vi "Untitled 2.vi"(6 "Axis":enum16{"X", "Y", "X+Y"}(ring), 7 "error IN":errorcluster, 10 "Data IN":T1={"App State"="", "Connect "=FALSE, "phandle out"=0, "Axis"=[], "S ramp"=30.0, "Acceleration"=100000.0, "Initial Speed"=10.0, "Normal Open / Close"=enum."Close", "Deceleration"=100000.0, "Creep"=30.0, "Speed"=1000.0, "X Axis"={"Operating State"="", "Current Position"=0.0, "Current Speed"=0.0, "Axis State"=0, "Angle"=0.0}, "Y Axis"={"Operating State"="", "Current Position"=0.0, "Current Speed"=0.0, "Axis State"=0, "Angle"=0.0}, "Distance"=0.0, "Direct of movement"=enum."Forward", "Move Method"=enum."Continue", "Move Mode"=enum."Relative", "Angle"=enum."0", "Times"=0, "Start Time"=0.0, "Step Flag"=FALSE, "x  dist"=[], "y dist"=[], "x angle array"=[], "y angle array"=[], "index"=0.0, "big motion angle"=0.0, "big angle"=[]}) -> (0 "error out":errorcluster, 3 "Data OUT":T1={"App State"="", "Connect "=FALSE, "phandle out"=0, "Axis"=[], "S ramp"=30.0, "Acceleration"=100000.0, "Initial Speed"=10.0, "Normal Open / Close"=enum."Close", "Deceleration"=100000.0, "Creep"=30.0, "Speed"=1000.0, "X Axis"={"Operating State"="", "Current Position"=0.0, "Current Speed"=0.0, "Axis State"=0, "Angle"=0.0}, "Y Axis"={"Operating State"="", "Current Position"=0.0, "Current Speed"=0.0, "Axis State"=0, "Angle"=0.0}, "Distance"=0.0, "Direct of movement"=enum."Forward", "Move Method"=enum."Continue", "Move Mode"=enum."Relative", "Angle"=enum."0", "Times"=0, "Start Time"=0.0, "Step Flag"=FALSE, "x  dist"=[], "y dist"=[], "x angle array"=[], "y angle array"=[], "index"=0.0, "big motion angle"=0.0, "big angle"=[]})   [LabVIEW 2015]
uses:
  Typedef/Data2.ctl
  zauxdll-2014/zauxdll.lvlib
panel:
  out "y angle array":i32[][](array[numeric])
  out "x angle array":i32[][](array[numeric])
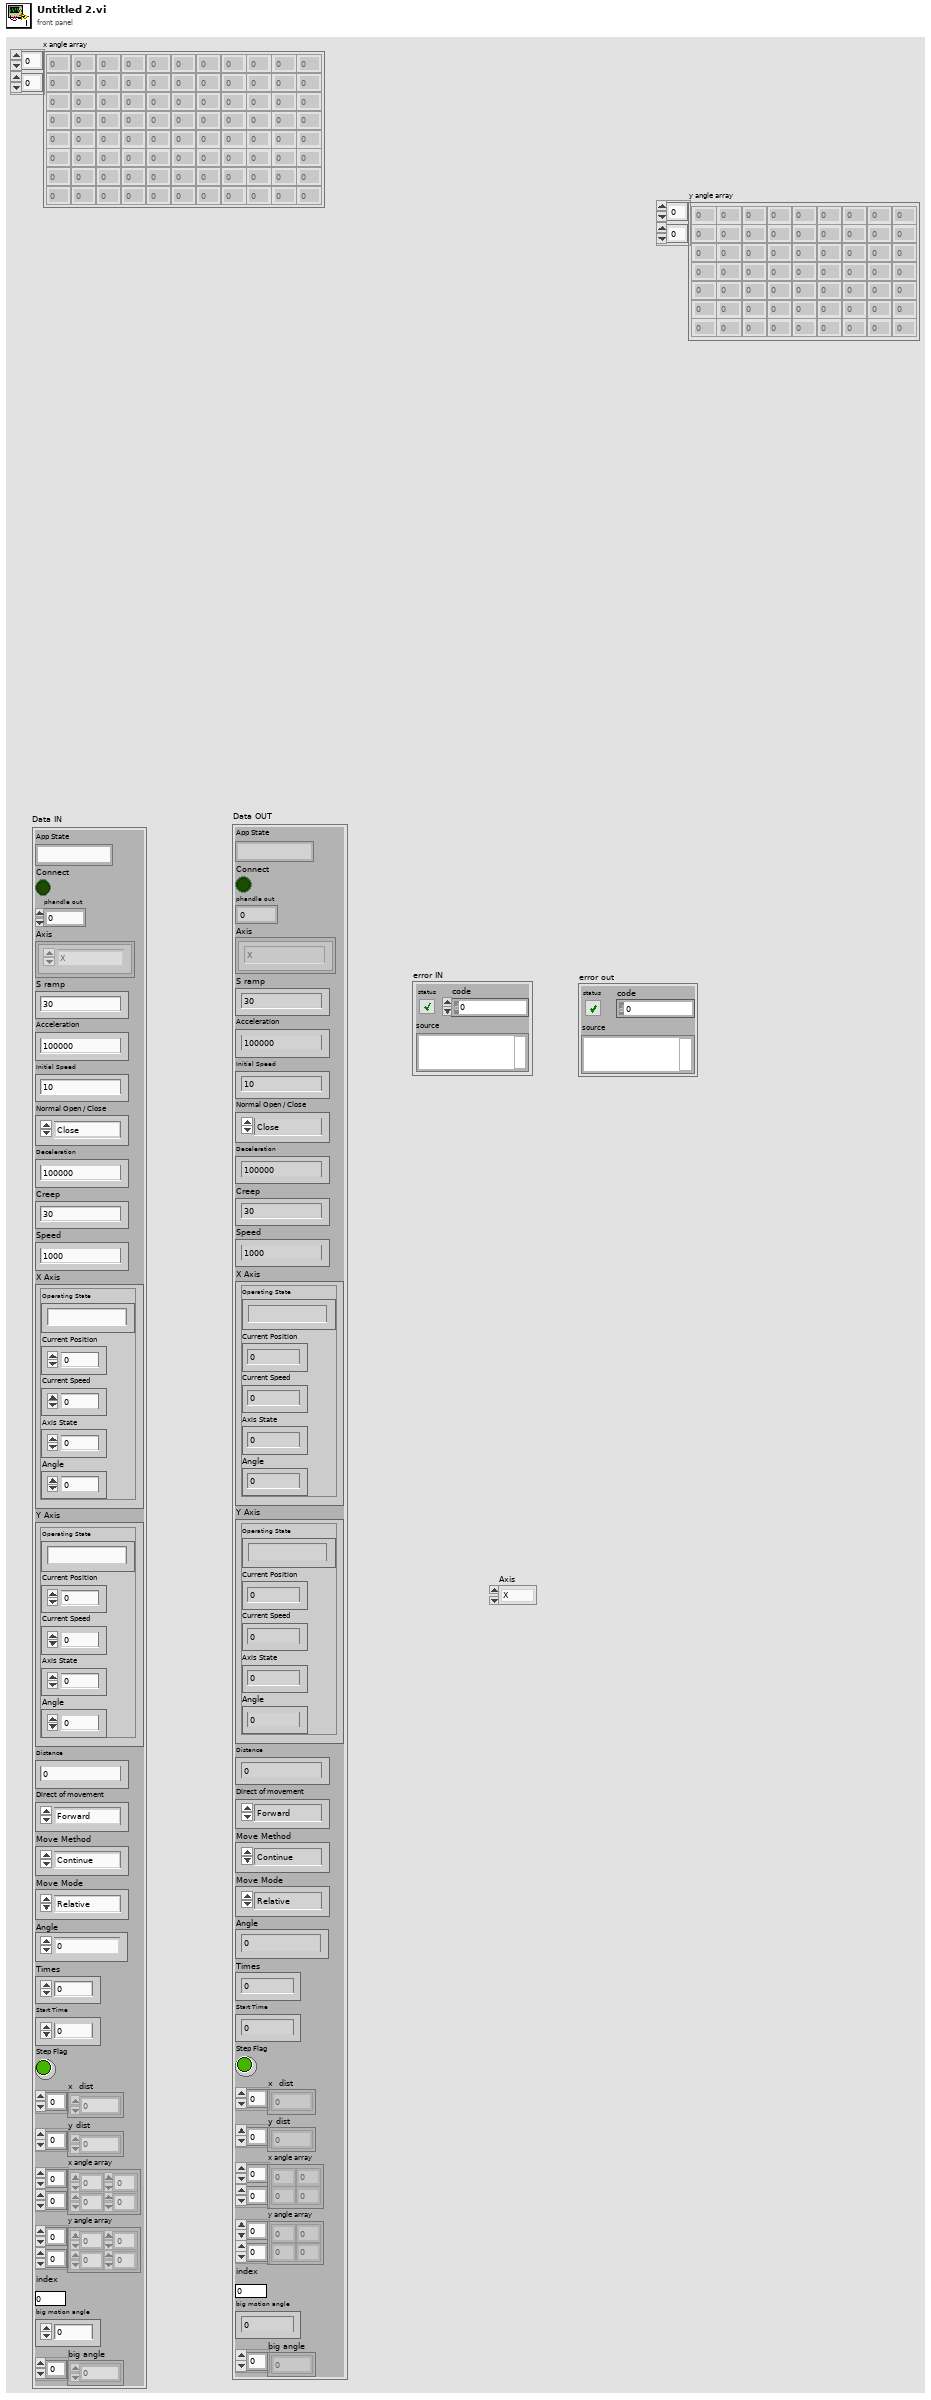
[diagram p1: front panel]
types:
  T1 = typedef "Data2.ctl" = cluster{"App State":string, "Connect ":bool, "phandle out":u32, "Axis":enum16{"X", "Y", "X+Y"}[], "S ramp":dbl, "Acceleration":dbl, "Initial Speed":dbl, "Normal Open / Close":enum16{"Open", "Close"}, "Deceleration":dbl, "Creep":dbl, "Speed":dbl, "X Axis":cluster{"Operating State":string, "Current Position":dbl, "Current Speed":dbl, "Axis State":i32, "Angle":dbl}, "Y Axis":cluster{"Operating State":string, "Current Position":dbl, "Current Speed":dbl, "Axis State":i32, "Angle":dbl}, "Distance":dbl, "Direct of movement":enum16{"Forward", "Backward"}, "Move Method":enum16{"Continue", "Inching"}, "Move Mode":enum16{"Relative", "Absolute"}, "Angle":enum32{"0", "1", "10", "30", "34", "60", "90", "180", "-1", "-10"}, "Times":i32, "Start Time":dbl, "Step Flag":bool, "x  dist":dbl[], "y dist":dbl[], "x angle array":i32[][], "y angle array":i32[][], "index":dbl, "big motion angle":dbl, "big angle":dbl[]}
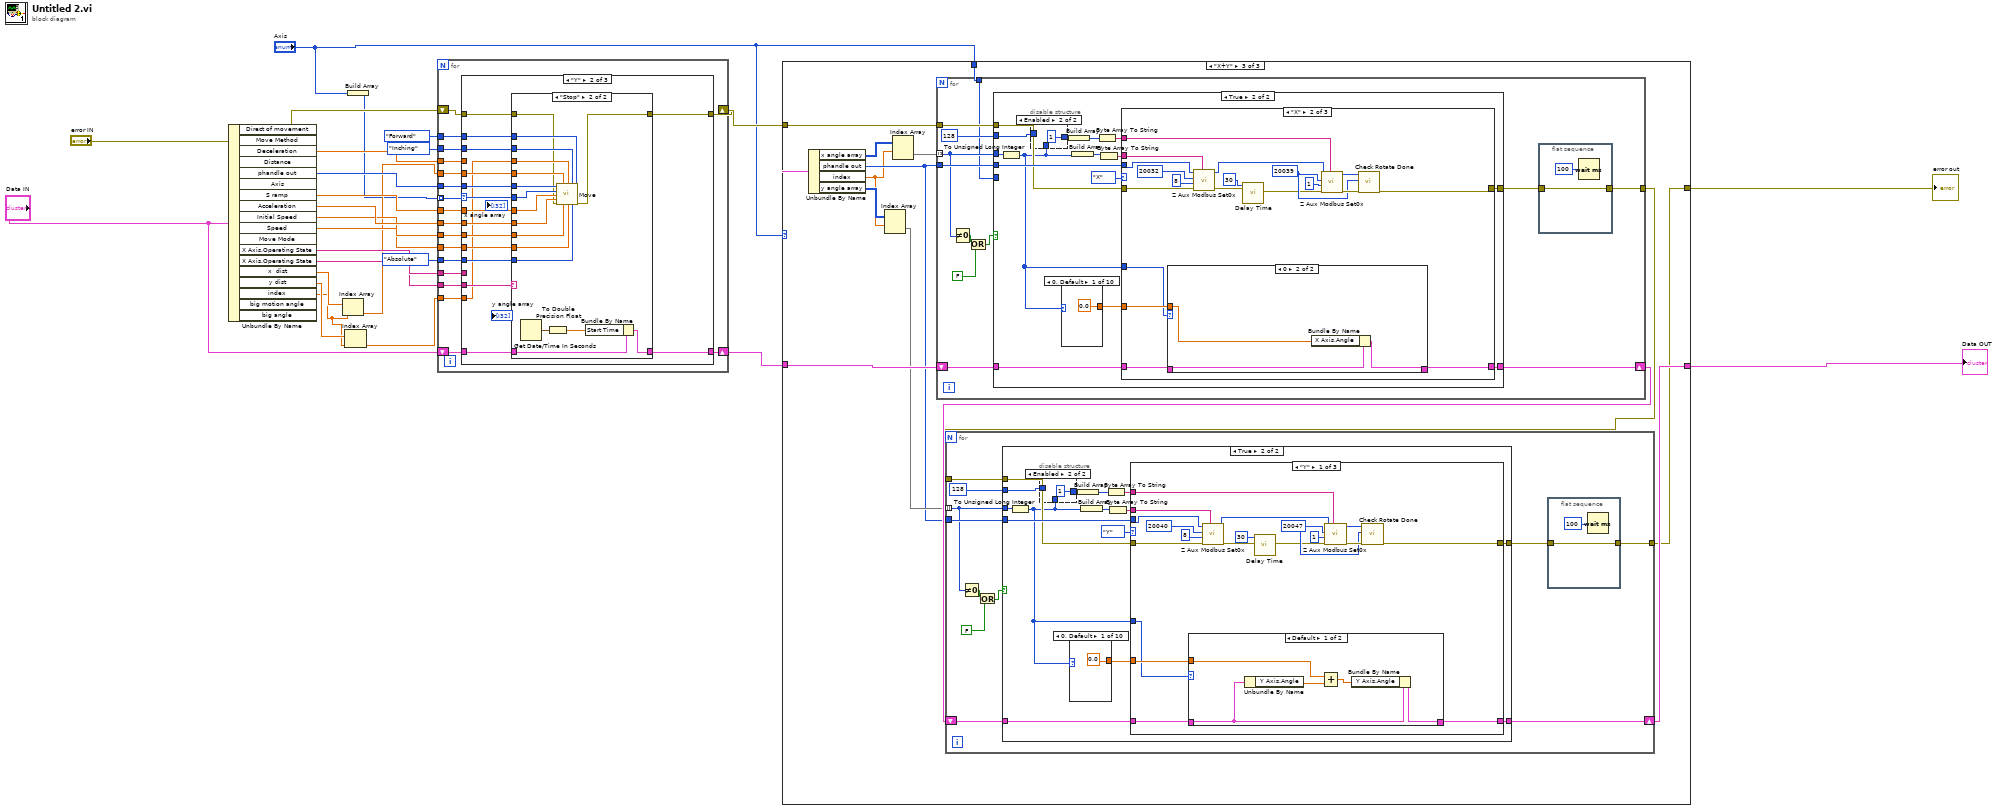
[diagram p0: block diagram]
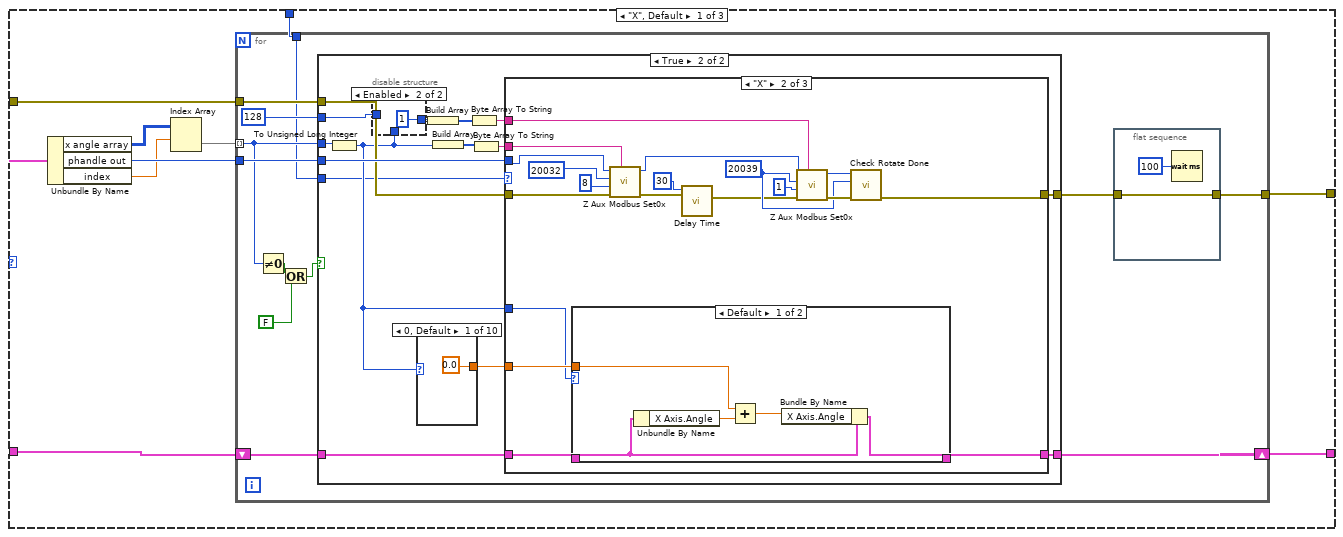
[diagram p2: hidden frame]
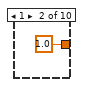
[diagram p4: hidden frame]
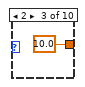
[diagram p5: hidden frame]
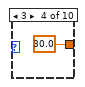
[diagram p6: hidden frame]
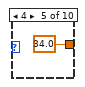
[diagram p7: hidden frame]
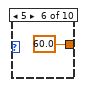
[diagram p8: hidden frame]
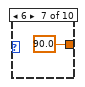
[diagram p9: hidden frame]
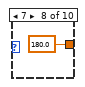
[diagram p10: hidden frame]
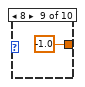
[diagram p11: hidden frame]
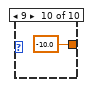
[diagram p12: hidden frame]
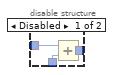
[diagram p13: hidden frame]
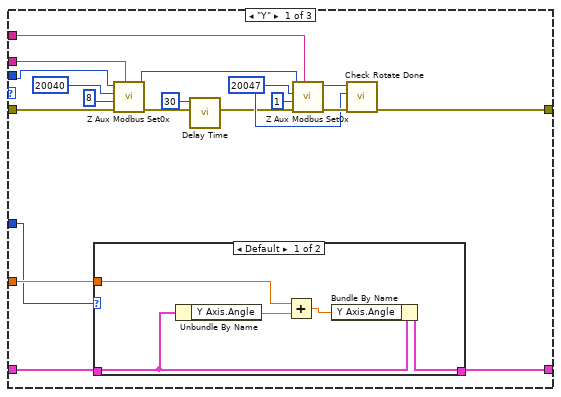
[diagram p14: hidden frame]
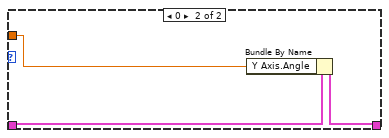
[diagram p15: hidden frame]
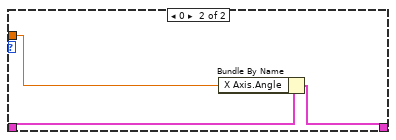
[diagram p16: hidden frame]
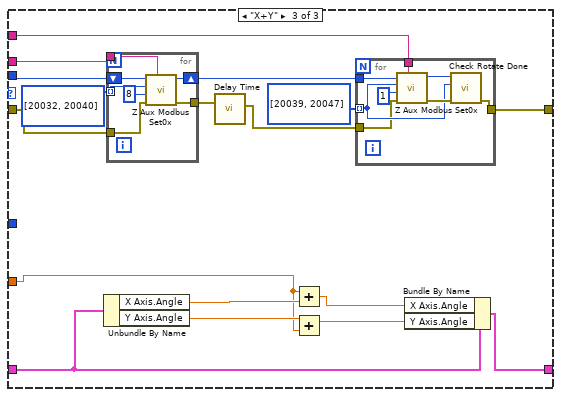
[diagram p17: hidden frame]
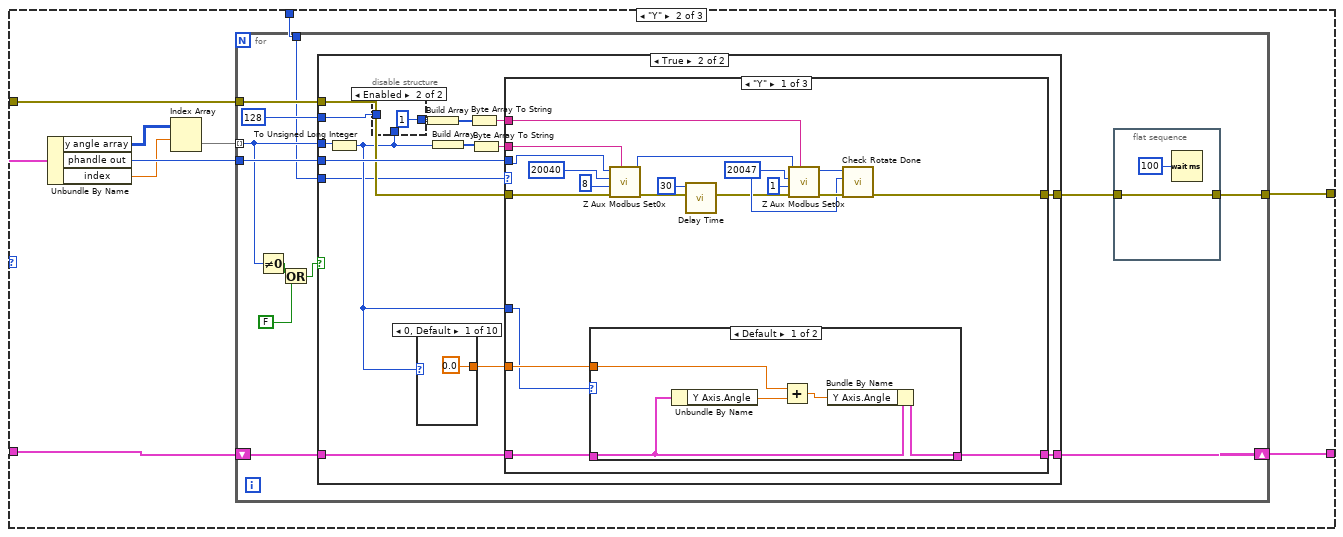
[diagram p18: hidden frame]
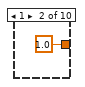
[diagram p20: hidden frame]
diagram:
  n1 = Unbundle By Name("Data IN") -> ("Deceleration"=w19:dbl, "phandle out"=w24:u32, "S ramp"=w23:dbl, "Acceleration"=w22:dbl, "Initial Speed"=w21:dbl, "Speed"=w20:dbl, "X Axis.Operating State"=w18:string, "X Axis.Operating State"=w17:string, "x  dist"=w10:dbl[], "y dist"=w3:dbl[], "index"=w2:dbl)  [unwired: 7 out]
  n2 = Index Array(array=w10, index=w2) -> (element=w6:dbl)
  n3 = Index Array(array=w3, index=w2) -> (element=w1:dbl)
  n4 = Build Array("Axis") -> (w5:enum16{"X", "Y", "X+Y"}[])
  n5 = for {
    tunnel: w24 -> [w42]
    tunnel: w23 -> [w41]
    tunnel: w22 -> [w40]
    tunnel: w21 -> [w39]
    tunnel: w20 -> [w38]
    tunnel: enum16{"Continue", "Inching"}."Inching" ("Move Method") -> [w37]
    tunnel: w19 -> [w36]
    tunnel: w5 -> [w35] mode=indexing
    tunnel: w6 -> [w34]
    tunnel: enum16{"Forward", "Backward"}."Forward" ("Direct of movement") -> [w33]
    tunnel: enum16{"Relative", "Absolute"}."Absolute" ("Move Mode") -> [w32]
    tunnel: w18 -> [w31]
    tunnel: w17 -> [w30]
    shift-right: [w28] -> w14
    shift-left: "Data IN" -> [w29]
    shift-right: [w26] -> w13
    shift-left: "error IN" -> [w27]
    tunnel: w1 -> [w25]
    n6 = case shown="\"Y\"" w35 {
      selector: w35 -> [w51 w87 _]
      tunnel: w42 -> [w58 w93 w134]
      tunnel: w41 -> [w57 w92 w133]
      tunnel: w40 -> [w56 w91 w132]
      tunnel: w39 -> [w55 w90 w131]
      tunnel: w38 -> [w54 w89 w130]
      tunnel: w37 -> [w53 w88 w129]
      tunnel: w36 -> [w52 _ w128]
      tunnel: w34 -> [w49 w85 w115]
      tunnel: w33 -> [w50 w86 w127]
      tunnel: w32 -> [w48 w84 w126]
      tunnel: w31 -> [w47 _ w125]
      tunnel: w30 -> [_ w83 w123]
      tunnel: w29 -> [w46 w82 w119]
      tunnel: [w45 w81 w118] -> w28
      tunnel: w27 -> [w44 w80 w117]
      tunnel: [w43 w79 w116] -> w26
      tunnel: w25 -> [_ w78 w114]
      frame "X", Default {
        n7 = case shown="\"Stop\"" w47 {
          tunnel: w58 -> [_ w77]
          tunnel: w57 -> [_ w76]
          tunnel: w56 -> [_ w75]
          tunnel: w55 -> [_ w74]
          tunnel: w54 -> [_ w73]
          tunnel: w53 -> [_ w72]
          tunnel: w52 -> [_ w71]
          tunnel: w51 -> [_ w70]
          tunnel: w50 -> [_ w69]
          tunnel: w49 -> [_ w68]
          tunnel: w48 -> [_ w67]
          tunnel: w46 -> [w60 w66]
          tunnel: [w60 w65] -> w45
          tunnel: w44 -> [w59 w62]
          tunnel: [w59 w61] -> w43
          frame "False", Default {
          }
          frame "Stop" {
            n8 = Get Date/Time In Seconds() -> (seconds since 1Jan1904=w64:timestamp)
            n9 = call "Move.vi"("handle"=w77, "Distance"=w68, "Decel"=w71, "Move Method"=w72, "Direct of movement"=w69, "Axis"=w70, "Sramp"=w76, "Accel"=w75, "error in (no error)"=w62, "Lspeed"=w74, "Speed"=w73, "Move Mode"=w67) -> ("error out"=w61:errorcluster)  [unwired: 3 in]
            n10 = To Double Precision Float(number=w64) -> (double precision float=w63:dbl)
            n11 = Bundle By Name(cluster=w66, "Start Time"=w63) -> (w65:T1)
          }
        }
      }
      frame "Y" {
        n12 = case shown="\"Stop\"" w83 {
          tunnel: w93 -> [_ w112]
          tunnel: w92 -> [_ w111]
          tunnel: w91 -> [_ w110]
          tunnel: w90 -> [_ w109]
          tunnel: w89 -> [_ w108]
          tunnel: w88 -> [_ w107]
          tunnel: w78 -> [_ w106]
          tunnel: w87 -> [_ w105]
          tunnel: w86 -> [_ w104]
          tunnel: w85 -> [_ w103]
          tunnel: w84 -> [_ w102]
          tunnel: w82 -> [w95 w99]
          tunnel: [w95 w98] -> w81
          tunnel: w80 -> [w94 w97]
          tunnel: [w94 w96] -> w79
          frame "False", Default {
          }
          frame "Stop" {
            n13 = Get Date/Time In Seconds() -> (seconds since 1Jan1904=w101:timestamp)
            n14 = To Double Precision Float(number=w101) -> (double precision float=w100:dbl)
            n15 = call "Move.vi"("handle"=w112, "Distance"=w103, "Decel"=w106, "Move Method"=w107, "Direct of movement"=w104, "Axis"=w105, "Sramp"=w111, "Accel"=w110, "error in (no error)"=w97, "Lspeed"=w109, "Speed"=w108, "Move Mode"=w102) -> ("error out"=w96:errorcluster)  [unwired: 3 in]
            n16 = Bundle By Name(cluster=w99, "Start Time"=w100) -> (w98:T1)
          }
        }
      }
      frame "X+Y" {
        w124 = "Stop" ("y")
        n17 = Build Array(w115, w114) -> (w113:dbl[])
        n18 = Equal?(x=w125, y=w124) -> (x = y?=w122:bool)
        n19 = Equal?(x=w124, y=w123) -> (x = y?=w120:bool)
        n20 = And(x=w122, y=w120) -> (x .and. y?=w121:bool)
        n21 = case shown="True" w121 {
          tunnel: w134 -> [_ w153]
          tunnel: w133 -> [_ w152]
          tunnel: w132 -> [_ w151]
          tunnel: w131 -> [_ w150]
          tunnel: w130 -> [_ w149]
          tunnel: w129 -> [_ w148]
          tunnel: w128 -> [_ w147]
          tunnel: w113 -> [_ w145]
          tunnel: w127 -> [_ w144]
          tunnel: w126 -> [_ w143]
          tunnel: w119 -> [w136 w142]
          tunnel: [w136 w141] -> w118
          tunnel: w117 -> [w135 w138]
          tunnel: [w135 w137] -> w116
          frame False {
          }
          frame True {
            n22 = Get Date/Time In Seconds() -> (seconds since 1Jan1904=w140:timestamp)
            n23 = To Double Precision Float(number=w140) -> (double precision float=w139:dbl)
            n24 = for {
              tunnel: w153 -> [w166]
              tunnel: w152 -> [w165]
              tunnel: w151 -> [w164]
              tunnel: w150 -> [w163]
              tunnel: w149 -> [w162]
              tunnel: w148 -> [w161]
              tunnel: w147 -> [w160]
              tunnel: i32[] [0, 1] -> [w159] mode=indexing
              tunnel: w145 -> [w158] mode=indexing
              tunnel: w144 -> [w157]
              tunnel: w143 -> [w156]
              tunnel: w138 -> [w155]
              tunnel: [w154] -> w137
              n25 = call "Move.vi"("handle"=w166, "Distance"=w158, "Decel"=w160, "Move Method"=w161, "Direct of movement"=w157, "Axis"=w159, "Sramp"=w165, "Accel"=w164, "error in (no error)"=w155, "Lspeed"=w163, "Speed"=w162, "Move Mode"=w156) -> ("error out"=w154:errorcluster)  [unwired: 3 in]
            }
            n26 = Bundle By Name(cluster=w142, "Start Time"=w139) -> (w141:T1)
          }
        }
      }
    }
  }
  n27 = case shown="\"X+Y\"" "Axis" {
    tunnel: w14 -> [w173 w313 w454]
    tunnel: w13 -> [w172 w312 w458]
    tunnel: [w171 w311 w450] -> w12
    tunnel: [w170 w310 w452] -> w11
    tunnel: "Axis" -> [w169 w309 w457]
    frame "X", Default {
      n28 = Unbundle By Name(w173) -> ("x angle array"=w168:i32[][], "phandle out"=w175:u32, "index"=w167:dbl)
      n29 = Index Array(array=w168, index (row)=w167) -> (element=w174:i32[])  [unwired: 1 in]
      n30 = for {
        tunnel: w175 -> [w183]
        tunnel: w172 -> [w187]
        tunnel: w174 -> [w182] mode=indexing
        shift-right: [w184] -> w170
        shift-left: w173 -> [w185]
        tunnel: [w178] -> w171
        tunnel: w169 -> [w176]
        n31 = Not Equal To 0?(x=w182) -> (x != 0?=w180:bool)
        n32 = Or(x=w180, y=FALSE) -> (x .or. y?=w181:bool)
        n33 = case shown="True" w181 {
          tunnel: w183 -> [_ w206]
          tunnel: w187 -> [w191 w205]
          tunnel: u32 128 -> [_ w204]
          tunnel: w185 -> [w190 w198]
          tunnel: w182 -> [_ w197]
          tunnel: [w190 w196] -> w184
          tunnel: [w191 w195] -> w179
          tunnel: w176 -> [_ w192]
          frame False {
          }
          frame True {
            n34 = To Unsigned Long Integer(number=w197) -> (unsigned 32bit integer=w193:u32)
            n35 = disable-structure shown="Enabled" {
              disable-tunnel: w204 -> [w219 _]
              disable-tunnel: [w218 u32 1] -> w203
              disable-tunnel: w193 -> [w217 _]
              frame Disabled {
                n36 = Add(x=w219, y=w217) -> (x+y=w218:u32)
              }
              frame Enabled {
              }
            }
            n37 = case shown="0, Default" w193 {
              tunnel: [0.0 1.0 10.0 30.0 34.0 60.0 90.0 180.0 -1.0 -10.0] -> w199
              frame 0, Default {
              }
              frame 1 {
              }
              frame 2 {
              }
              frame 3 {
              }
              frame 4 {
              }
              frame 5 {
              }
              frame 6 {
              }
              frame 7 {
              }
              frame 8 {
              }
              frame 9 {
              }
            }
            n38 = Build Array(w203) -> (w202:u32[])
            n39 = Build Array(w193) -> (w194:u32[])
            n40 = Byte Array To String(unsigned byte array=w202) -> (string=w201:string)
            n41 = Byte Array To String(unsigned byte array=w194) -> (string=w200:string)
            n42 = case shown="\"X\"" w192 {
              tunnel: w206 -> [w236 w263 w290]
              tunnel: w201 -> [w237 w264 w291]
              tunnel: w200 -> [w235 w262 w289]
              tunnel: w205 -> [w230 w257 w286]
              tunnel: [w225 w252 w282] -> w195
              tunnel: w198 -> [w224 w251 w279]
              tunnel: [w223 w250 w278] -> w196
              tunnel: w199 -> [w222 w249 w275]
              tunnel: w193 -> [w221 w248 _]
              frame "Y" {
                w231 = u16 20047 ("start")
                n43 = case shown="Default" w221 {
                  tunnel: w224 -> [w244 w247]
                  tunnel: [w243 w246] -> w223
                  tunnel: w222 -> [w240 w245]
                  frame Default {
                    n44 = Unbundle By Name(w244) -> ("Y Axis.Angle"=w241:dbl)
                    n45 = Add(x=w240, y=w241) -> (x+y=w242:dbl)
                    n46 = Bundle By Name(cluster=w244, "Y Axis.Angle"=w242) -> (w243:T1)
                  }
                  frame 0 {
                    n47 = Bundle By Name(cluster=w247, "Y Axis.Angle"=w245) -> (w246:T1)
                  }
                }
                n48 = call "Z Aux Modbus Set0x.vi"("pdata"=w235, "error in (no error)"=w230, "inum"=u16 8, "start"=u16 20040, "handle"=w236) -> ("error out"=w228:errorcluster, "handle out"=w229:u32)  [unwired: 3 in, 2 out]
                n49 = call "Delay Time.vi"("error in (no error)"=w228, "Delay(ms)"=u32 30) -> ("error out"=w226:errorcluster)  [unwired: 9 in]
                n50 = call "Z Aux Modbus Set0x.vi"("pdata"=w237, "error in (no error)"=w226, "inum"=u16 1, "start"=w231, "handle"=w229) -> ("error out"=w239:errorcluster, "handle out"=w238:u32)  [unwired: 3 in, 2 out]
                n51 = call "Check Rotate Done.vi"("error in (no error)"=w239, "start"=w231, "phandle in"=w238) -> ("error out"=w225:errorcluster)  [unwired: 8 in]
              }
              frame "X" {
                w258 = u16 20039 ("start")
                n52 = case shown="Default" w248 {
                  tunnel: w251 -> [w271 w274]
                  tunnel: [w270 w273] -> w250
                  tunnel: w249 -> [w267 w272]
                  frame Default {
                    n53 = Unbundle By Name(w271) -> ("X Axis.Angle"=w269:dbl)
                    n54 = Add(x=w267, y=w269) -> (x+y=w268:dbl)
                    n55 = Bundle By Name(cluster=w271, "X Axis.Angle"=w268) -> (w270:T1)
                  }
                  frame 0 {
                    n56 = Bundle By Name(cluster=w274, "X Axis.Angle"=w272) -> (w273:T1)
                  }
                }
                n57 = call "Z Aux Modbus Set0x.vi"("pdata"=w262, "error in (no error)"=w257, "inum"=u16 8, "start"=u16 20032, "handle"=w263) -> ("error out"=w255:errorcluster, "handle out"=w256:u32)  [unwired: 3 in, 2 out]
                n58 = call "Delay Time.vi"("error in (no error)"=w255, "Delay(ms)"=u32 30) -> ("error out"=w253:errorcluster)  [unwired: 9 in]
                n59 = call "Z Aux Modbus Set0x.vi"("pdata"=w264, "error in (no error)"=w253, "inum"=u16 1, "start"=w258, "handle"=w256) -> ("error out"=w266:errorcluster, "handle out"=w265:u32)  [unwired: 3 in, 2 out]
                n60 = call "Check Rotate Done.vi"("error in (no error)"=w266, "start"=w258, "phandle in"=w265) -> ("error out"=w252:errorcluster)  [unwired: 8 in]
              }
              frame "X+Y" {
                n61 = Unbundle By Name(w279) -> ("X Axis.Angle"=w281:dbl, "Y Axis.Angle"=w280:dbl)
                n62 = for {
                  tunnel: w289 -> [w305]
                  shift-right: [w304] -> w284
                  shift-left: w290 -> [w306]
                  tunnel: i32[] [20032, 20040] -> [w302] mode=indexing
                  tunnel: w286 -> [w301]
                  tunnel: [w300] -> w285
                  n63 = call "Z Aux Modbus Set0x.vi"("pdata"=w305, "error in (no error)"=w301, "inum"=u16 8, "start"=w302, "handle"=w306) -> ("error out"=w300:errorcluster, "handle out"=w304:u32)  [unwired: 3 in, 2 out]
                }
                n64 = call "Delay Time.vi"("error in (no error)"=w285) -> ("error out"=w283:errorcluster)  [unwired: 10 in]
                n65 = Add(x=w275, y=w281) -> (x+y=w277:dbl)
                n66 = Add(x=w280, y=w275) -> (x+y=w276:dbl)
                n67 = for {
                  tunnel: w291 -> [w297]
                  tunnel: w284 -> [w296]
                  tunnel: i32[] [20039, 20047] -> [w294] mode=indexing
                  tunnel: w283 -> [w293]
                  tunnel: [w292] -> w282
                  n68 = call "Z Aux Modbus Set0x.vi"("pdata"=w297, "error in (no error)"=w293, "inum"=u16 1, "start"=w294, "handle"=w296) -> ("error out"=w299:errorcluster, "handle out"=w298:u32)  [unwired: 3 in, 2 out]
                  n69 = call "Check Rotate Done.vi"("error in (no error)"=w299, "start"=w294, "phandle in"=w298) -> ("error out"=w292:errorcluster)  [unwired: 8 in]
                }
                n70 = Bundle By Name(cluster=w279, "X Axis.Angle"=w277, "Y Axis.Angle"=w276) -> (w278:T1)
              }
            }
          }
        }
        n71 = flat-sequence {
          tunnel: w179 -> [w189]
          tunnel: [w189] -> w178
          frame #0 {
            n72 = Wait (ms)(milliseconds to wait=u32 100) -> ()  [unwired: 1 out]
          }
        }
      }
    }
    frame "Y" {
      n73 = Unbundle By Name(w313) -> ("y angle array"=w308:i32[][], "phandle out"=w315:u32, "index"=w307:dbl)
      n74 = Index Array(array=w308, index (row)=w307) -> (element=w314:i32[])  [unwired: 1 in]
      n75 = for {
        tunnel: w315 -> [w323]
        tunnel: w312 -> [w327]
        tunnel: w314 -> [w322] mode=indexing
        shift-right: [w324] -> w310
        shift-left: w313 -> [w325]
        tunnel: [w318] -> w311
        tunnel: w309 -> [w316]
        n76 = Not Equal To 0?(x=w322) -> (x != 0?=w320:bool)
        n77 = Or(x=w320, y=FALSE) -> (x .or. y?=w321:bool)
        n78 = case shown="True" w321 {
          tunnel: w323 -> [_ w346]
          tunnel: w327 -> [w331 w345]
          tunnel: u32 128 -> [_ w344]
          tunnel: w325 -> [w330 w338]
          tunnel: w322 -> [_ w337]
          tunnel: [w330 w336] -> w324
          tunnel: [w331 w335] -> w319
          tunnel: w316 -> [_ w332]
          frame False {
          }
          frame True {
            n79 = To Unsigned Long Integer(number=w337) -> (unsigned 32bit integer=w333:u32)
            n80 = disable-structure shown="Enabled" {
              disable-tunnel: w344 -> [w359 _]
              disable-tunnel: [w358 u32 1] -> w343
              disable-tunnel: w333 -> [w357 _]
              frame Disabled {
                n81 = Add(x=w359, y=w357) -> (x+y=w358:u32)
              }
              frame Enabled {
              }
            }
            n82 = case shown="0, Default" w333 {
              tunnel: [0.0 1.0 10.0 30.0 34.0 60.0 90.0 180.0 -1.0 -10.0] -> w339
              frame 0, Default {
              }
              frame 1 {
              }
              frame 2 {
              }
              frame 3 {
              }
              frame 4 {
              }
              frame 5 {
              }
              frame 6 {
              }
              frame 7 {
              }
              frame 8 {
              }
              frame 9 {
              }
            }
            n83 = Build Array(w343) -> (w342:u32[])
            n84 = Build Array(w333) -> (w334:u32[])
            n85 = Byte Array To String(unsigned byte array=w342) -> (string=w341:string)
            n86 = Byte Array To String(unsigned byte array=w334) -> (string=w340:string)
            n87 = case shown="\"Y\"" w332 {
              tunnel: w346 -> [w376 w403 w430]
              tunnel: w341 -> [w377 w404 w431]
              tunnel: w340 -> [w375 w402 w429]
              tunnel: w345 -> [w370 w397 w426]
              tunnel: [w365 w392 w422] -> w335
              tunnel: w338 -> [w364 w391 w419]
              tunnel: [w363 w390 w418] -> w336
              tunnel: w339 -> [w362 w389 w415]
              tunnel: w333 -> [w361 w388 _]
              frame "Y" {
                w371 = u16 20047 ("start")
                n88 = case shown="Default" w361 {
                  tunnel: w364 -> [w384 w387]
                  tunnel: [w383 w386] -> w363
                  tunnel: w362 -> [w380 w385]
                  frame Default {
                    n89 = Unbundle By Name(w384) -> ("Y Axis.Angle"=w381:dbl)
                    n90 = Add(x=w380, y=w381) -> (x+y=w382:dbl)
                    n91 = Bundle By Name(cluster=w384, "Y Axis.Angle"=w382) -> (w383:T1)
                  }
                  frame 0 {
                    n92 = Bundle By Name(cluster=w387, "Y Axis.Angle"=w385) -> (w386:T1)
                  }
                }
                n93 = call "Z Aux Modbus Set0x.vi"("pdata"=w375, "error in (no error)"=w370, "inum"=u16 8, "start"=u16 20040, "handle"=w376) -> ("error out"=w368:errorcluster, "handle out"=w369:u32)  [unwired: 3 in, 2 out]
                n94 = call "Delay Time.vi"("error in (no error)"=w368, "Delay(ms)"=u32 30) -> ("error out"=w366:errorcluster)  [unwired: 9 in]
                n95 = call "Z Aux Modbus Set0x.vi"("pdata"=w377, "error in (no error)"=w366, "inum"=u16 1, "start"=w371, "handle"=w369) -> ("error out"=w379:errorcluster, "handle out"=w378:u32)  [unwired: 3 in, 2 out]
                n96 = call "Check Rotate Done.vi"("error in (no error)"=w379, "start"=w371, "phandle in"=w378) -> ("error out"=w365:errorcluster)  [unwired: 8 in]
              }
              frame "X" {
                w398 = u16 20039 ("start")
                n97 = case shown="0" w388 {
                  tunnel: w391 -> [w411 w414]
                  tunnel: [w410 w413] -> w390
                  tunnel: w389 -> [w407 w412]
                  frame Default {
                    n98 = Unbundle By Name(w411) -> ("X Axis.Angle"=w409:dbl)
                    n99 = Add(x=w407, y=w409) -> (x+y=w408:dbl)
                    n100 = Bundle By Name(cluster=w411, "X Axis.Angle"=w408) -> (w410:T1)
                  }
                  frame 0 {
                    n101 = Bundle By Name(cluster=w414, "X Axis.Angle"=w412) -> (w413:T1)
                  }
                }
                n102 = call "Z Aux Modbus Set0x.vi"("pdata"=w402, "error in (no error)"=w397, "inum"=u16 8, "start"=u16 20032, "handle"=w403) -> ("error out"=w395:errorcluster, "handle out"=w396:u32)  [unwired: 3 in, 2 out]
                n103 = call "Delay Time.vi"("error in (no error)"=w395, "Delay(ms)"=u32 30) -> ("error out"=w393:errorcluster)  [unwired: 9 in]
                n104 = call "Z Aux Modbus Set0x.vi"("pdata"=w404, "error in (no error)"=w393, "inum"=u16 1, "start"=w398, "handle"=w396) -> ("error out"=w406:errorcluster, "handle out"=w405:u32)  [unwired: 3 in, 2 out]
                n105 = call "Check Rotate Done.vi"("error in (no error)"=w406, "start"=w398, "phandle in"=w405) -> ("error out"=w392:errorcluster)  [unwired: 8 in]
              }
              frame "X+Y" {
                n106 = Unbundle By Name(w419) -> ("X Axis.Angle"=w421:dbl, "Y Axis.Angle"=w420:dbl)
                n107 = for {
                  tunnel: w429 -> [w445]
                  shift-right: [w444] -> w424
                  shift-left: w430 -> [w446]
                  tunnel: i32[] [20032, 20040] -> [w442] mode=indexing
                  tunnel: w426 -> [w441]
                  tunnel: [w440] -> w425
                  n108 = call "Z Aux Modbus Set0x.vi"("pdata"=w445, "error in (no error)"=w441, "inum"=u16 8, "start"=w442, "handle"=w446) -> ("error out"=w440:errorcluster, "handle out"=w444:u32)  [unwired: 3 in, 2 out]
                }
                n109 = call "Delay Time.vi"("error in (no error)"=w425) -> ("error out"=w423:errorcluster)  [unwired: 10 in]
                n110 = Add(x=w415, y=w421) -> (x+y=w417:dbl)
                n111 = Add(x=w420, y=w415) -> (x+y=w416:dbl)
                n112 = for {
                  tunnel: w431 -> [w437]
                  tunnel: w424 -> [w436]
                  tunnel: i32[] [20039, 20047] -> [w434] mode=indexing
                  tunnel: w423 -> [w433]
                  tunnel: [w432] -> w422
                  n113 = call "Z Aux Modbus Set0x.vi"("pdata"=w437, "error in (no error)"=w433, "inum"=u16 1, "start"=w434, "handle"=w436) -> ("error out"=w439:errorcluster, "handle out"=w438:u32)  [unwired: 3 in, 2 out]
                  n114 = call "Check Rotate Done.vi"("error in (no error)"=w439, "start"=w434, "phandle in"=w438) -> ("error out"=w432:errorcluster)  [unwired: 8 in]
                }
                n115 = Bundle By Name(cluster=w419, "X Axis.Angle"=w417, "Y Axis.Angle"=w416) -> (w418:T1)
              }
            }
          }
        }
        n116 = flat-sequence {
          tunnel: w319 -> [w329]
          tunnel: [w329] -> w318
          frame #0 {
            n117 = Wait (ms)(milliseconds to wait=u32 100) -> ()  [unwired: 1 out]
          }
        }
      }
    }
    frame "X+Y" {
      n118 = Unbundle By Name(w454) -> ("x angle array"=w456:i32[][], "phandle out"=w448:u32, "index"=w447:dbl, "y angle array"=w455:i32[][])
      n119 = Index Array(array=w455, index (row)=w447) -> (element=w449:i32[])  [unwired: 1 in]
      n120 = Index Array(array=w456, index (row)=w447) -> (element=w459:i32[])  [unwired: 1 in]
      n121 = for {
        tunnel: w448 -> [w598]
        tunnel: w458 -> [w601]
        tunnel: w459 -> [w597] mode=indexing
        shift-right: [w591] -> w453
        shift-left: w454 -> [w599]
        tunnel: [w590] -> w451
        tunnel: w457 -> [w592]
        n122 = Not Equal To 0?(x=w597) -> (x != 0?=w595:bool)
        n123 = Or(x=w595, y=FALSE) -> (x .or. y?=w596:bool)
        n124 = case shown="True" w596 {
          tunnel: w598 -> [_ w620]
          tunnel: w601 -> [w605 w619]
          tunnel: u32 128 -> [_ w618]
          tunnel: w599 -> [w604 w612]
          tunnel: w597 -> [_ w611]
          tunnel: [w604 w610] -> w591
          tunnel: [w605 w609] -> w594
          tunnel: w592 -> [_ _]
          frame False {
          }
          frame True {
            n125 = To Unsigned Long Integer(number=w611) -> (unsigned 32bit integer=w607:u32)
            n126 = disable-structure shown="Enabled" {
              disable-tunnel: w618 -> [w633 _]
              disable-tunnel: [w632 u32 1] -> w617
              disable-tunnel: w607 -> [w631 _]
              frame Disabled {
                n127 = Add(x=w633, y=w631) -> (x+y=w632:u32)
              }
              frame Enabled {
              }
            }
            n128 = case shown="0, Default" w607 {
              tunnel: [0.0 1.0 10.0 30.0 34.0 60.0 90.0 180.0 -1.0 -10.0] -> w613
              frame 0, Default {
              }
              frame 1 {
              }
              frame 2 {
              }
              frame 3 {
              }
              frame 4 {
              }
              frame 5 {
              }
              frame 6 {
              }
              frame 7 {
              }
              frame 8 {
              }
              frame 9 {
              }
            }
            n129 = Build Array(w617) -> (w616:u32[])
            n130 = Build Array(w607) -> (w608:u32[])
            n131 = Byte Array To String(unsigned byte array=w616) -> (string=w615:string)
            n132 = Byte Array To String(unsigned byte array=w608) -> (string=w614:string)
            n133 = case shown="\"X\"" enum16{"X", "Y", "X+Y"}."X" ("Axis") {
              tunnel: w620 -> [w650 w677 w704]
              tunnel: w615 -> [w651 w678 w705]
              tunnel: w614 -> [w649 w676 w703]
              tunnel: w619 -> [w644 w671 w700]
              tunnel: [w639 w666 w696] -> w609
              tunnel: w612 -> [w638 w665 w693]
              tunnel: [w637 w664 w692] -> w610
              tunnel: w613 -> [w636 w663 w689]
              tunnel: w607 -> [w635 w662 _]
              frame "Y" {
                w645 = u16 20047 ("start")
                n134 = case shown="0" w635 {
                  tunnel: w638 -> [w658 w661]
                  tunnel: [w657 w660] -> w637
                  tunnel: w636 -> [w654 w659]
                  frame Default {
                    n135 = Unbundle By Name(w658) -> ("X Axis.Angle"=w655:dbl)
                    n136 = Add(x=w654, y=w655) -> (x+y=w656:dbl)
                    n137 = Bundle By Name(cluster=w658, "X Axis.Angle"=w656) -> (w657:T1)
                  }
                  frame 0 {
                    n138 = Bundle By Name(cluster=w661, "X Axis.Angle"=w659) -> (w660:T1)
                  }
                }
                n139 = call "Z Aux Modbus Set0x.vi"("pdata"=w649, "error in (no error)"=w644, "inum"=u16 8, "start"=u16 20040, "handle"=w650) -> ("error out"=w642:errorcluster, "handle out"=w643:u32)  [unwired: 3 in, 2 out]
                n140 = call "Delay Time.vi"("error in (no error)"=w642, "Delay(ms)"=u32 30) -> ("error out"=w640:errorcluster)  [unwired: 9 in]
                n141 = call "Z Aux Modbus Set0x.vi"("pdata"=w651, "error in (no error)"=w640, "inum"=u16 1, "start"=w645, "handle"=w643) -> ("error out"=w653:errorcluster, "handle out"=w652:u32)  [unwired: 3 in, 2 out]
                n142 = call "Check Rotate Done.vi"("error in (no error)"=w653, "start"=w645, "phandle in"=w652) -> ("error out"=w639:errorcluster)  [unwired: 8 in]
              }
              frame "X" {
                w672 = u16 20039 ("start")
                n143 = case shown="0" w662 {
                  tunnel: w665 -> [w685 w688]
                  tunnel: [w684 w687] -> w664
                  tunnel: w663 -> [w681 w686]
                  frame Default {
                    n144 = Unbundle By Name(w685) -> ("X Axis.Angle"=w683:dbl)
                    n145 = Add(x=w681, y=w683) -> (x+y=w682:dbl)
                    n146 = Bundle By Name(cluster=w685, "X Axis.Angle"=w682) -> (w684:T1)
                  }
                  frame 0 {
                    n147 = Bundle By Name(cluster=w688, "X Axis.Angle"=w686) -> (w687:T1)
                  }
                }
                n148 = call "Z Aux Modbus Set0x.vi"("pdata"=w676, "error in (no error)"=w671, "inum"=u16 8, "start"=u16 20032, "handle"=w677) -> ("error out"=w669:errorcluster, "handle out"=w670:u32)  [unwired: 3 in, 2 out]
                n149 = call "Delay Time.vi"("error in (no error)"=w669, "Delay(ms)"=u32 30) -> ("error out"=w667:errorcluster)  [unwired: 9 in]
                n150 = call "Z Aux Modbus Set0x.vi"("pdata"=w678, "error in (no error)"=w667, "inum"=u16 1, "start"=w672, "handle"=w670) -> ("error out"=w680:errorcluster, "handle out"=w679:u32)  [unwired: 3 in, 2 out]
                n151 = call "Check Rotate Done.vi"("error in (no error)"=w680, "start"=w672, "phandle in"=w679) -> ("error out"=w666:errorcluster)  [unwired: 8 in]
              }
              frame "X+Y" {
                n152 = Unbundle By Name(w693) -> ("X Axis.Angle"=w695:dbl, "Y Axis.Angle"=w694:dbl)
                n153 = for {
                  tunnel: w703 -> [w719]
                  shift-right: [w718] -> w698
                  shift-left: w704 -> [w720]
                  tunnel: i32[] [20032, 20040] -> [w716] mode=indexing
                  tunnel: w700 -> [w715]
                  tunnel: [w714] -> w699
                  n154 = call "Z Aux Modbus Set0x.vi"("pdata"=w719, "error in (no error)"=w715, "inum"=u16 8, "start"=w716, "handle"=w720) -> ("error out"=w714:errorcluster, "handle out"=w718:u32)  [unwired: 3 in, 2 out]
                }
                n155 = call "Delay Time.vi"("error in (no error)"=w699) -> ("error out"=w697:errorcluster)  [unwired: 10 in]
                n156 = Add(x=w689, y=w695) -> (x+y=w691:dbl)
                n157 = Add(x=w694, y=w689) -> (x+y=w690:dbl)
                n158 = for {
                  tunnel: w705 -> [w711]
                  tunnel: w698 -> [w710]
                  tunnel: i32[] [20039, 20047] -> [w708] mode=indexing
                  tunnel: w697 -> [w707]
                  tunnel: [w706] -> w696
                  n159 = call "Z Aux Modbus Set0x.vi"("pdata"=w711, "error in (no error)"=w707, "inum"=u16 1, "start"=w708, "handle"=w710) -> ("error out"=w713:errorcluster, "handle out"=w712:u32)  [unwired: 3 in, 2 out]
                  n160 = call "Check Rotate Done.vi"("error in (no error)"=w713, "start"=w708, "phandle in"=w712) -> ("error out"=w706:errorcluster)  [unwired: 8 in]
                }
                n161 = Bundle By Name(cluster=w693, "X Axis.Angle"=w691, "Y Axis.Angle"=w690) -> (w692:T1)
              }
            }
          }
        }
        n162 = flat-sequence {
          tunnel: w594 -> [w603]
          tunnel: [w603] -> w590
          frame #0 {
            n163 = Wait (ms)(milliseconds to wait=u32 100) -> ()  [unwired: 1 out]
          }
        }
      }
      n164 = for {
        tunnel: w448 -> [w466]
        tunnel: w451 -> [w470]
        tunnel: w449 -> [w465] mode=indexing
        shift-right: [w467] -> w452
        shift-left: w453 -> [w468]
        tunnel: [w461] -> w450
        n165 = Not Equal To 0?(x=w465) -> (x != 0?=w463:bool)
        n166 = Or(x=w463, y=FALSE) -> (x .or. y?=w464:bool)
        n167 = case shown="True" w464 {
          tunnel: w466 -> [_ w489]
          tunnel: w470 -> [w474 w488]
          tunnel: u32 128 -> [_ w487]
          tunnel: w468 -> [w473 w481]
          tunnel: w465 -> [_ w480]
          tunnel: [w473 w479] -> w467
          tunnel: [w474 w478] -> w462
          frame False {
          }
          frame True {
            n168 = To Unsigned Long Integer(number=w480) -> (unsigned 32bit integer=w476:u32)
            n169 = disable-structure shown="Enabled" {
              disable-tunnel: w487 -> [w502 _]
              disable-tunnel: [w501 u32 1] -> w486
              disable-tunnel: w476 -> [w500 _]
              frame Disabled {
                n170 = Add(x=w502, y=w500) -> (x+y=w501:u32)
              }
              frame Enabled {
              }
            }
            n171 = case shown="0, Default" w476 {
              tunnel: [0.0 1.0 10.0 30.0 34.0 60.0 90.0 180.0 -1.0 -10.0] -> w482
              frame 0, Default {
              }
              frame 1 {
              }
              frame 2 {
              }
              frame 3 {
              }
              frame 4 {
              }
              frame 5 {
              }
              frame 6 {
              }
              frame 7 {
              }
              frame 8 {
              }
              frame 9 {
              }
            }
            n172 = Build Array(w486) -> (w485:u32[])
            n173 = Build Array(w476) -> (w477:u32[])
            n174 = Byte Array To String(unsigned byte array=w485) -> (string=w484:string)
            n175 = Byte Array To String(unsigned byte array=w477) -> (string=w483:string)
            n176 = case shown="\"Y\"" enum16{"X", "Y", "X+Y"}."Y" ("Axis") {
              tunnel: w489 -> [w519 w546 w573]
              tunnel: w484 -> [w520 w547 w574]
              tunnel: w483 -> [w518 w545 w572]
              tunnel: w488 -> [w513 w540 w569]
              tunnel: [w508 w535 w565] -> w478
              tunnel: w481 -> [w507 w534 w562]
              tunnel: [w506 w533 w561] -> w479
              tunnel: w482 -> [w505 w532 w558]
              tunnel: w476 -> [w504 w531 _]
              frame "Y" {
                w514 = u16 20047 ("start")
                n177 = case shown="Default" w504 {
                  tunnel: w507 -> [w527 w530]
                  tunnel: [w526 w529] -> w506
                  tunnel: w505 -> [w523 w528]
                  frame Default {
                    n178 = Unbundle By Name(w527) -> ("Y Axis.Angle"=w524:dbl)
                    n179 = Add(x=w523, y=w524) -> (x+y=w525:dbl)
                    n180 = Bundle By Name(cluster=w527, "Y Axis.Angle"=w525) -> (w526:T1)
                  }
                  frame 0 {
                    n181 = Bundle By Name(cluster=w530, "Y Axis.Angle"=w528) -> (w529:T1)
                  }
                }
                n182 = call "Z Aux Modbus Set0x.vi"("pdata"=w518, "error in (no error)"=w513, "inum"=u16 8, "start"=u16 20040, "handle"=w519) -> ("error out"=w511:errorcluster, "handle out"=w512:u32)  [unwired: 3 in, 2 out]
                n183 = call "Delay Time.vi"("error in (no error)"=w511, "Delay(ms)"=u32 30) -> ("error out"=w509:errorcluster)  [unwired: 9 in]
                n184 = call "Z Aux Modbus Set0x.vi"("pdata"=w520, "error in (no error)"=w509, "inum"=u16 1, "start"=w514, "handle"=w512) -> ("error out"=w522:errorcluster, "handle out"=w521:u32)  [unwired: 3 in, 2 out]
                n185 = call "Check Rotate Done.vi"("error in (no error)"=w522, "start"=w514, "phandle in"=w521) -> ("error out"=w508:errorcluster)  [unwired: 8 in]
              }
              frame "X" {
                w541 = u16 20039 ("start")
                n186 = case shown="0" w531 {
                  tunnel: w534 -> [w554 w557]
                  tunnel: [w553 w556] -> w533
                  tunnel: w532 -> [w550 w555]
                  frame Default {
                    n187 = Unbundle By Name(w554) -> ("X Axis.Angle"=w552:dbl)
                    n188 = Add(x=w550, y=w552) -> (x+y=w551:dbl)
                    n189 = Bundle By Name(cluster=w554, "X Axis.Angle"=w551) -> (w553:T1)
                  }
                  frame 0 {
                    n190 = Bundle By Name(cluster=w557, "X Axis.Angle"=w555) -> (w556:T1)
                  }
                }
                n191 = call "Z Aux Modbus Set0x.vi"("pdata"=w545, "error in (no error)"=w540, "inum"=u16 8, "start"=u16 20032, "handle"=w546) -> ("error out"=w538:errorcluster, "handle out"=w539:u32)  [unwired: 3 in, 2 out]
                n192 = call "Delay Time.vi"("error in (no error)"=w538, "Delay(ms)"=u32 30) -> ("error out"=w536:errorcluster)  [unwired: 9 in]
                n193 = call "Z Aux Modbus Set0x.vi"("pdata"=w547, "error in (no error)"=w536, "inum"=u16 1, "start"=w541, "handle"=w539) -> ("error out"=w549:errorcluster, "handle out"=w548:u32)  [unwired: 3 in, 2 out]
                n194 = call "Check Rotate Done.vi"("error in (no error)"=w549, "start"=w541, "phandle in"=w548) -> ("error out"=w535:errorcluster)  [unwired: 8 in]
              }
              frame "X+Y" {
                n195 = Unbundle By Name(w562) -> ("X Axis.Angle"=w564:dbl, "Y Axis.Angle"=w563:dbl)
                n196 = for {
                  tunnel: w572 -> [w588]
                  shift-right: [w587] -> w567
                  shift-left: w573 -> [w589]
                  tunnel: i32[] [20032, 20040] -> [w585] mode=indexing
                  tunnel: w569 -> [w584]
                  tunnel: [w583] -> w568
                  n197 = call "Z Aux Modbus Set0x.vi"("pdata"=w588, "error in (no error)"=w584, "inum"=u16 8, "start"=w585, "handle"=w589) -> ("error out"=w583:errorcluster, "handle out"=w587:u32)  [unwired: 3 in, 2 out]
                }
                n198 = call "Delay Time.vi"("error in (no error)"=w568) -> ("error out"=w566:errorcluster)  [unwired: 10 in]
                n199 = Add(x=w558, y=w564) -> (x+y=w560:dbl)
                n200 = Add(x=w563, y=w558) -> (x+y=w559:dbl)
                n201 = for {
                  tunnel: w574 -> [w580]
                  tunnel: w567 -> [w579]
                  tunnel: i32[] [20039, 20047] -> [w577] mode=indexing
                  tunnel: w566 -> [w576]
                  tunnel: [w575] -> w565
                  n202 = call "Z Aux Modbus Set0x.vi"("pdata"=w580, "error in (no error)"=w576, "inum"=u16 1, "start"=w577, "handle"=w579) -> ("error out"=w582:errorcluster, "handle out"=w581:u32)  [unwired: 3 in, 2 out]
                  n203 = call "Check Rotate Done.vi"("error in (no error)"=w582, "start"=w577, "phandle in"=w581) -> ("error out"=w575:errorcluster)  [unwired: 8 in]
                }
                n204 = Bundle By Name(cluster=w562, "X Axis.Angle"=w560, "Y Axis.Angle"=w559) -> (w561:T1)
              }
            }
          }
        }
        n205 = flat-sequence {
          tunnel: w462 -> [w472]
          tunnel: [w472] -> w461
          frame #0 {
            n206 = Wait (ms)(milliseconds to wait=u32 100) -> ()  [unwired: 1 out]
          }
        }
      }
    }
  }
  "error out" <- w12
  "Data OUT" <- w11
